vi "lab3.vi"() -> ()   [LabVIEW 2020]
doc: "Use this template to build a master/slave design pattern. The master loop always executes. It notifies one or more slave loops to execute their code. The slave loop(s) continue executing until they complete, then wait for another notification. Contrast this with the Producer/Consumer pattern in which the consumer loops execute only when they have data in their queue."
uses:
  <vilib>/Utility/miscctls.llb/LVPositionTypeDef.ctl
panel:
  out "Position":cluster{"Left":dbl, "Top":dbl}
  in  "Tab Control":enum32{"Visualisation", "Plots"}(tab)
  out "Beam":bool
  in  "stop":bool
  out "Event":bool
  out "Beam Positon Detector 1 - x axis":dbl[](graph)
  out "Beam Positon Detector 1 - y axis":dbl[](graph)
  out "Beam Positon Detector 2 - x axis":dbl[](graph)
  out "Beam Positon Detector 2 - y axis":dbl[](graph)
  out "Beam Positon Detector 3 - x axis":dbl[](graph)
  out "Beam Positon Detector 3 - y axis":dbl[](graph)
  out "Particles momentum":dbl[](graph)
  # "Source of image: http://sps.web.cern.ch/sps/"
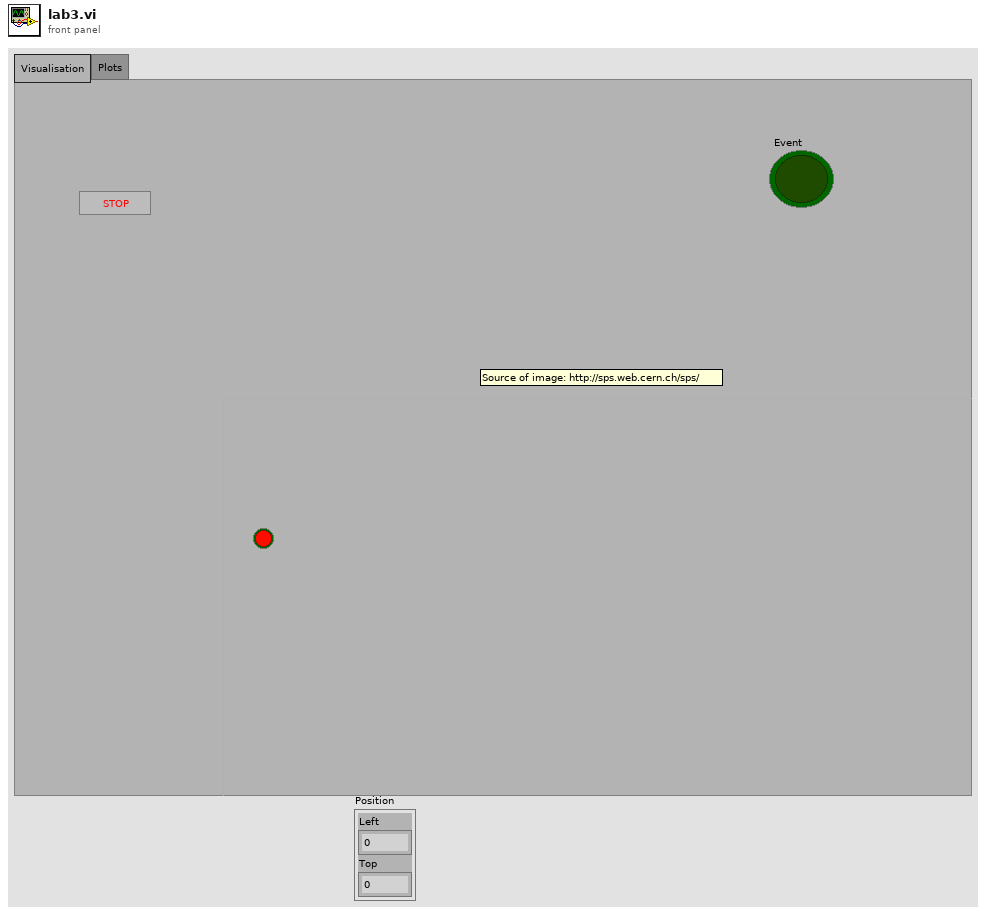
[diagram p1: front panel]
types:
  T1 = enum8{"Enabled", "Disabled", "Disabled and Grayed Out"}
  T2 = typedef "LVPositionTypeDef.ctl" = cluster{"Left":i32, "Top":i32}
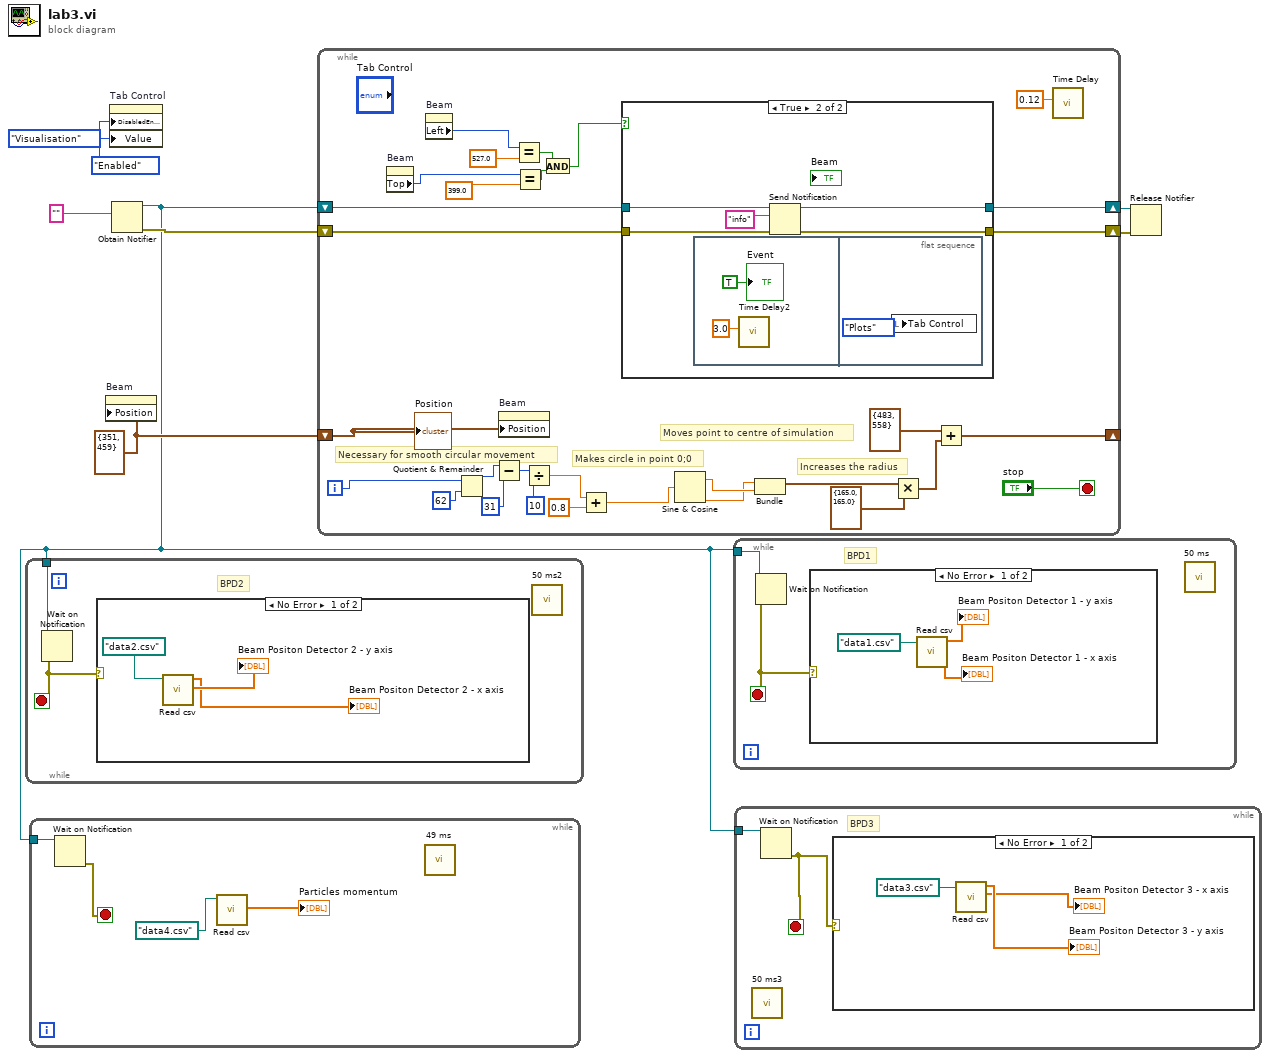
[diagram p0: block diagram]
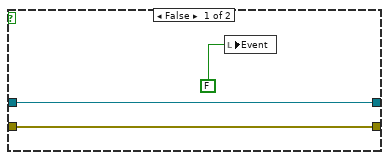
[diagram p5: hidden frame]
diagram:
  w4 = T2 {"Left"=351, "Top"=459} ("Position")
  n1 = property on="Beam" class="Bool (strict)"("Position"=w4) -> ()  [unwired: 2 in, 2 out]
  n2 = property on="Tab Control" class="TabCtl (strict)"("DisabledEnum"=T1."Enabled" ("Disabled"), "Value"=enum32{"Visualisation", "Plots"}."Visualisation" ("Tab Control")) -> ()  [unwired: 2 in, 2 out]
  n3 = Obtain Notifier(notification data type="") -> (notifier out=w2:refnum<notifier>, error out=w7:errorcluster)  [unwired: 3 in, 1 out]
  n4 = while {
    tunnel: w2 -> [w10]
    stop <- w9 stop-if-true
    # "BPD2"
    n5 = Wait on Notification(notifier=w10) -> (error out=w9:errorcluster)  [unwired: 3 in, 3 out]
    n6 = case shown="No Error" w9 {
      frame No Error {
        n7 = call "Read csv.vi"("name or relative path"=path "data2.csv") -> ("Array 2"=→"Beam Positon Detector 2 - y axis":dbl[], "Array"=→"Beam Positon Detector 2 - x axis":dbl[])  [unwired: 9 in]
      }
      frame Error {
      }
    }
    n8 = call "50 ms2"() -> ()  [unwired: 11 in, 1 out]
  }
  n9 = while {
    tunnel: w2 -> [w17]
    stop <- w16 stop-if-true
    n10 = Wait on Notification(notifier=w17) -> (error out=w16:errorcluster)  [unwired: 3 in, 3 out]
    n11 = call "Read csv.vi"("name or relative path"=path "data4.csv") -> ("Array 2"=→"Particles momentum":dbl[])  [unwired: 9 in, 1 out]
    n12 = call "49 ms"() -> ()  [unwired: 11 in, 1 out]
  }
  n13 = while {
    shift-right: [w46] -> w8
    shift-left: w2 -> [w45]
    shift-right: [w43] -> w6
    shift-left: w7 -> [w44]
    shift-right: [w27] -> _
    shift-left: w4 -> [w26]
    i -> [w31]
    stop <- "stop" stop-if-true
    # "Necessary for smooth circular movement"
    # "Increases the radius"
    # "Moves point to centre of simulation"
    # "Makes circle in point 0;0"
    n14 = property on="Beam" class="Bool (strict)"() -> ("Top"=w22:i32)  [unwired: 2 in, 2 out]
    n15 = property on="Beam" class="Bool (strict)"() -> ("Left"=w23:i32)  [unwired: 2 in, 2 out]
    n16 = Quotient & Remainder(x=w31, y=62) -> (x-y*floor(x/y)=w32:i32)  [unwired: 1 out]
    n17 = Subtract(x=w32, y=31) -> (x-y=w33:i32)
    n18 = property on="Beam" class="Bool (strict)"("Position"=w26) -> ()  [unwired: 2 in, 2 out]
    n19 = Equal?(x=w23, y=527.0) -> (x = y?=w21:bool)
    n20 = Equal?(x=w22, y=399.0) -> (x = y?=w20:bool)
    n21 = Divide(x=w33, y=10) -> (x/y=w29:dbl)
    n22 = And(x=w21, y=w20) -> (x .and. y?=w19:bool)
    n23 = Add(x=w29, y=0.8) -> (x+y=w28:dbl)
    n24 = case shown="True" w19 {
      tunnel: [w50 w54] -> w46
      tunnel: w45 -> [w50 w55]
      tunnel: w44 -> [w49 w53]
      tunnel: [w49 w52] -> w43
      frame False {
        n25 = local write "Event"(FALSE ("Event")) -> ()
      }
      frame True {
        n26 = flat-sequence {
          frame #0 {
            n27 = call "Time Delay2"("Delay Time (s)"=3.0) -> ()  [unwired: 10 in, 1 out]
            "Event" <- TRUE ("Event")
          }
          frame #1 {
            n28 = local write "Tab Control"(enum32{"Visualisation", "Plots"}."Plots" ("Tab Control")) -> ()
          }
        }
        n29 = Send Notification(notification="info", notifier=w55, error in (no error)=w53) -> (notifier out=w54:refnum<notifier>, error out=w52:errorcluster)
      }
    }
    n30 = Sine & Cosine(0:w28) -> (1:w38:dbl, 2:w37:dbl)
    n31 = Bundle(w37, w38) -> (w42:cluster{dbl, dbl})  [unwired: 1 in]
    n32 = Multiply(x=w42, y=cluster{dbl, dbl} {165.0, 165.0}) -> (x*y=w39:cluster{dbl, dbl})
    n33 = Add(x=T2 {"Left"=483, "Top"=558} ("Position"), y=w39) -> (x+y=w27:cluster{dbl, dbl})
    n34 = call "Time Delay"("Delay Time (s)"=0.12) -> ()  [unwired: 10 in, 1 out]
    "Position" <- w26
  }
  n35 = while {
    tunnel: w2 -> [w60]
    stop <- w59 stop-if-true
    # "BPD1"
    n36 = Wait on Notification(notifier=w60) -> (error out=w59:errorcluster)  [unwired: 3 in, 3 out]
    n37 = case shown="No Error" w59 {
      frame No Error {
        n38 = call "Read csv.vi"("name or relative path"=path "data1.csv") -> ("Array 2"=→"Beam Positon Detector 1 - x axis":dbl[], "Array"=→"Beam Positon Detector 1 - y axis":dbl[])  [unwired: 9 in]
      }
      frame Error {
      }
    }
    n39 = call "50 ms"() -> ()  [unwired: 11 in, 1 out]
  }
  n40 = while {
    tunnel: w2 -> [w65]
    stop <- w64 stop-if-true
    # "BPD3"
    n41 = call "50 ms3"() -> ()  [unwired: 11 in, 1 out]
    n42 = Wait on Notification(notifier=w65) -> (error out=w64:errorcluster)  [unwired: 3 in, 3 out]
    n43 = case shown="No Error" w64 {
      frame No Error {
        n44 = call "Read csv.vi"("name or relative path"=path "data3.csv") -> ("Array 2"=→"Beam Positon Detector 3 - x axis":dbl[], "Array"=→"Beam Positon Detector 3 - y axis":dbl[])  [unwired: 9 in]
      }
      frame Error {
      }
    }
  }
  n45 = Release Notifier(notifier=w8, error in (no error)=w6) -> ()  [unwired: 1 in, 3 out]
